vi "Untitled 7 (SubVI).vi"(0 "Gaussianed cached Memory":refnum<k21>, 1 "Output Line Count 2":i16, 2 "Memory Out in":refnum<k21>, 3 "pixel cached Memory":refnum<k21>, 5 "DV in":bool, 7 "Output Line Count":i16, 9 "Width":u32, 12 "Height":u32, 13 "Data Out":fxp<+,12,12>, 14 "DelayRowCount":i16) -> (4 "addressInMemory":u32, 6 "data Out":fxp<+/-,13,13>, 8 "DV out":bool)   [LabVIEW 2016]
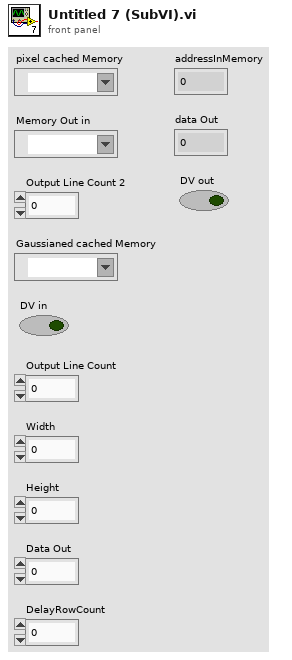
[diagram p1: front panel]
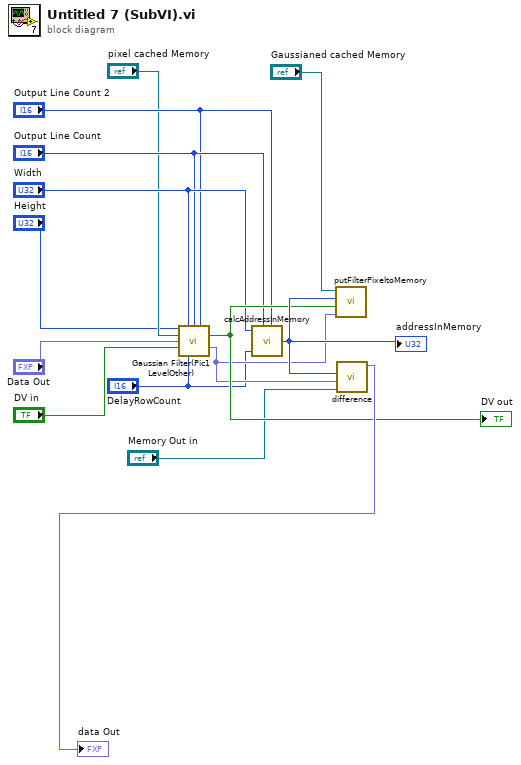
[diagram p0: block diagram]
diagram:
  n1 = call "Gaussian Filter(Pic1 LevelOther).vi"("Height"="Height", "Width"="Width", "Rows"="Output Line Count", "Cols"="Output Line Count 2", "Memory in"="pixel cached Memory", "Data in"="Data Out", "DV in"="DV in", "DelayRowCount"="DelayRowCount") -> ("DV out"=w12:bool, "Data Out"=w7:fxp<+,12,12>)  [unwired: 6 in]
  "DV out" <- w12
  n2 = call "calcAddressInMemory.vi"("Width"="Width", "Rows"="Output Line Count", "delayRowCount"="DelayRowCount", "Cols"="Output Line Count 2") -> ("addressInMemory"=w14:u32)  [unwired: 5 in]
  "addressInMemory" <- w14
  n3 = call "putFilterPixeltoMemory.vi"("Data In"=w7, "DV in"=w12, "addressInMemory"=w14, "Memory in"="Gaussianed cached Memory") -> ()
  n4 = call "difference.vi"("prePicMemory"="Memory Out in", "curPixel"=w7, "addressInMemory"=w14) -> ("data Out"=→"data Out":fxp<+/-,13,13>)  [unwired: 8 in]
